vi "GetNodeData__slk_msxml.vi"(0 "document in":refnum<class "msxml document.lvclass">, 5 "node in":refnum<class "msxml node.lvclass">, 11 "error in (no error)":errorcluster) -> (4 "document out":refnum<class "msxml document.lvclass">, 6 "node out":refnum<class "msxml node.lvclass">, 8 "node data":T1, 15 "error out":errorcluster)   [LabVIEW 2020, in "MSXML.lvlib" / "msxml node.lvclass"]
doc: "Returns the node date(name, text, and attributes) of MSXML Node."
uses:
  msxml node.lvclass
  MSXML Document/msxml document.lvclass
  Type Definition/NodeData__slk_msxml.ctl
  Type Definition/Attributes__slk_msxml.ctl
  Type Definition/Attribute__slk_msxml.ctl
  MSXML.lvlib
panel:
  # "GetNodeData__slk_msxml.vi\n\nReturns the node date(name, text, and attributes) of MSXML Node.\n\nNOTICE -- YOU MUST LEAVE THIS NOTICE IN PLACE.\n\nCopyright (c) 2004-2010 Shawn Liu <shawn.liu.cn@gmail.com>\n\nAll rights reserved."
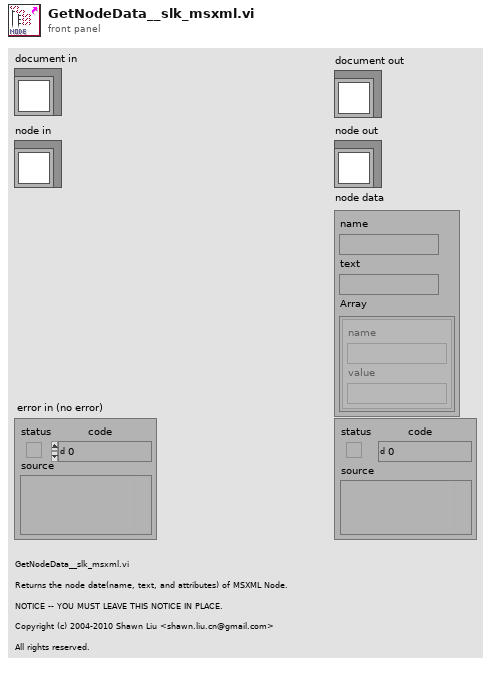
[diagram p1: front panel]
types:
  T1 = typedef "MSXML.lvlib/NodeData__slk_msxml.ctl" = cluster{"name":string, "text":string, "Array":T2}
  T2 = typedef "MSXML.lvlib/Attributes__slk_msxml.ctl" = T3[]
  T3 = typedef "MSXML.lvlib/Attribute__slk_msxml.ctl" = cluster{"name":string, "value":string}
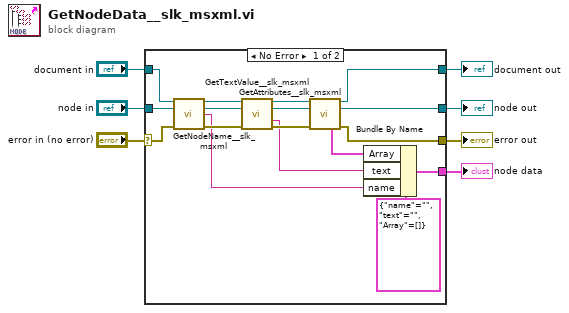
[diagram p0: block diagram]
diagram:
  n1 = case shown="No Error" "error in (no error)" {
    selector: "error in (no error)" -> [w16 w27]
    tunnel: [w15 w27] -> w4
    tunnel: [w10 w26] -> w6
    tunnel: "node in" -> [w23 w26]
    tunnel: "document in" -> [w24 w25]
    tunnel: [w9 w25] -> w2
    tunnel: [w11 _] -> w1
    frame No Error {
      n2 = call "GetNodeName__slk_msxml.vi"("document in"=w24, "node in"=w23, "error in (no error)"=w16) -> ("document out"=w22:refnum<class "msxml document.lvclass">, "node out"=w21:refnum<class "msxml node.lvclass">, "node name"=w12:string, "error out"=w18:errorcluster)  [unwired: 9 in]
      n3 = call "GetTextValue__slk_msxml.vi"("document in"=w22, "node in"=w21, "error in (no error)"=w18) -> ("document out"=w20:refnum<class "msxml document.lvclass">, "node out"=w19:refnum<class "msxml node.lvclass">, "text value"=w8:string, "error out"=w17:errorcluster)  [unwired: 9 in]
      n4 = call "GetAttributes__slk_msxml.vi"("document in"=w20, "node in"=w19, "error in (no error)"=w17) -> ("document out"=w9:refnum<class "msxml document.lvclass">, "node out"=w10:refnum<class "msxml node.lvclass">, "attributes"=w13:T2, "error out"=w15:errorcluster)  [unwired: 9 in]
      n5 = Bundle By Name(cluster=T1 {"name"="", "text"="", "Array"=[]} ("node data"), "Array"=w13, "text"=w8, "name"=w12) -> (w11:T1)
    }
    frame Error {
    }
  }
  "node out" <- w6
  "error out" <- w4
  "node data" <- w1
  "document out" <- w2
